vi "Acquire.vi"(0 "Hardware Resources in":T2 {"Baudrate" items=["110", "300", "600", "1200", "2400", "4800", "9600", "14400", "19200", "38400", "57600", "115200", "128000", "256000"]}, 7 "Data Queue Processing":T1, 9 "Data Queue Logging":T1, 11 "error in (no error)":errorcluster) -> (4 "Hardware Resources out":T2 {"Baudrate" items=["110", "300", "600", "1200", "2400", "4800", "9600", "14400", "19200", "38400", "57600", "115200", "128000", "256000"]}, 15 "error out":errorcluster)   [LabVIEW 2021, in "IMU Acquisition.lvlib"]
doc: "Perform the acquisition. Replace the contents of this diagram with calls to acquisition hardware."
uses:
  IMU Acquisition.lvlib
  Hardware Configuration.ctl
  Settings/baudrates.ctl
  IMU Data Queue.ctl
  IMU TimeDataStruct.ctl
  Settings/IMU Settings.lvlib
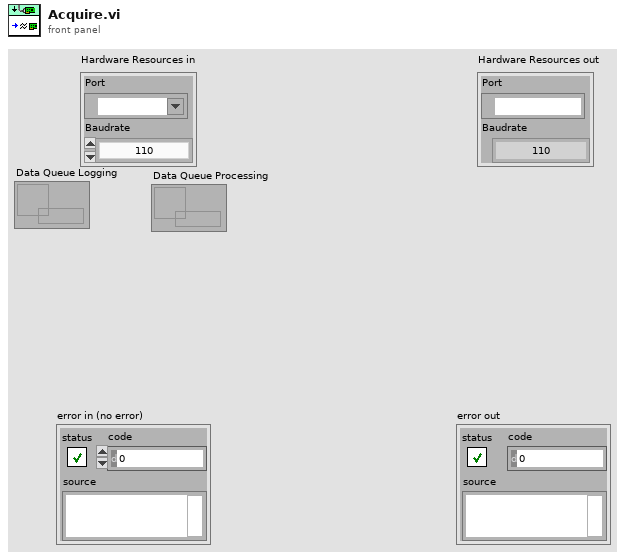
[diagram p1: front panel]
types:
  T1 = typedef "IMU Data Queue.ctl" = refnum<queue>
  T2 = typedef "IMU Acquisition.lvlib/Hardware Configuration.ctl" = cluster{"Port":refnum<visa-resource-name>, "Baudrate":T3}
  T3 = typedef "IMU Settings.lvlib/baudrates.ctl" = u16
  T4 = typedef "IMU TimeDataStruct.ctl" = cluster{string, dbl[]}
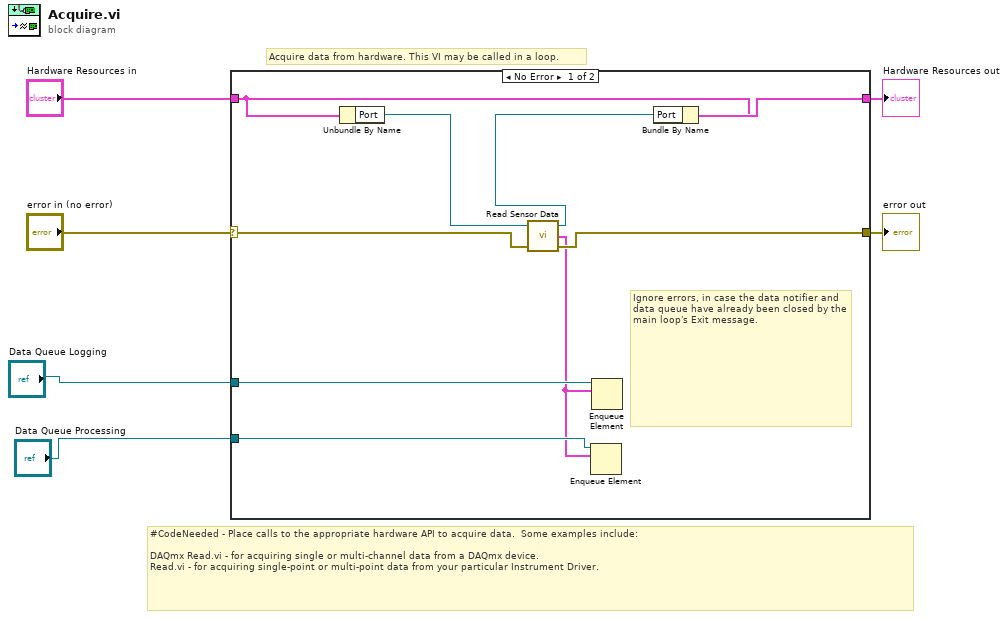
[diagram p0: block diagram]
diagram:
  # "Acquire data from hardware. This VI may be called in a loop."
  # "#CodeNeeded - Place calls to the appropriate hardware API to acquire data.  Some examples include:\n\nDAQmx Read.vi - for acquiring single or multi-channel data from a DAQmx device.\nRead.vi - for acquiring single-point or multi-point data from your particular Instrument Driver."
  n1 = case shown="No Error" "error in (no error)" {
    selector: "error in (no error)" -> [w10 w16]
    tunnel: [w9 w16] -> w5
    tunnel: "Hardware Resources in" -> [w14 w17]
    tunnel: [w15 w17] -> w3
    tunnel: "Data Queue Logging" -> [w13 _]
    tunnel: "Data Queue Processing" -> [w8 _]
    frame No Error {
      # "Ignore errors, in case the data notifier and data queue have already been closed by the main loop's Exit message."
      n2 = Unbundle By Name(w14) -> ("Port"=w12:refnum<visa-resource-name>)
      n3 = call "Read Sensor Data.vi"("error in (no error)"=w10, "VISA resource name"=w12) -> ("error out"=w9:errorcluster, "Data out"=w7:T4, "VISA resource name out"=w11:refnum<visa-resource-name>)  [unwired: 1 in]
      n4 = Enqueue Element(queue=w8, element=w7) -> ()  [unwired: 2 in, 3 out]
      n5 = Enqueue Element(queue=w13, element=w7) -> ()  [unwired: 2 in, 3 out]
      n6 = Bundle By Name(cluster=w14, "Port"=w11) -> (w15:T2)
    }
    frame Error {
    }
  }
  "Hardware Resources out" <- w3
  "error out" <- w5
